vi "names.vi"() -> ()   [LabVIEW 2012]
panel:
  in  "Frisbee Path":string[](array[string])
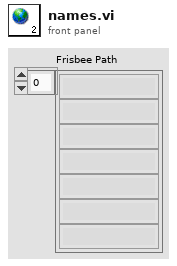
[diagram p1: front panel]
diagram:
